vi "Write.vi"(2 "Element":T1, 3 "timeout in ms (-1)":i32, 4 "Close (F)":bool) -> (7 "EnclaveChannel":T2, 8 "Closed?":bool, 9 "timed out?":bool)   [LabVIEW 2022 SP3, in "Enclave.lvlib"]
doc: "Writes values directly to the Channel Wire. How the value is transferred will depend on what readers are connected to the Channel Wire. Writes will typically return quickly unless there are size bounded lossless readers attached to the Channel Wire that cause writes to block until those readers have space available."
uses:
  Enclave.lvlib
  ))Channel.ctl
  Element.ctl
  Operation.ctl
  Enclave/Enclave.lvclass/Enclave.ctl
  Enclave/Check Ready.vi
  Enclave/Enclave.lvclass
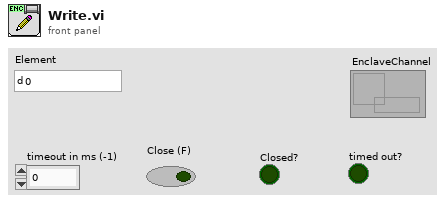
[diagram p1: front panel]
types:
  T1 = typedef "Enclave.lvlib/Element.ctl" = dbl
  T2 = typedef "Enclave.lvlib/))Channel.ctl" = refnum<queue>
  T3 = typedef "Enclave.lvlib/Operation.ctl" = enum16{"Get Core", "Init", "Close"}
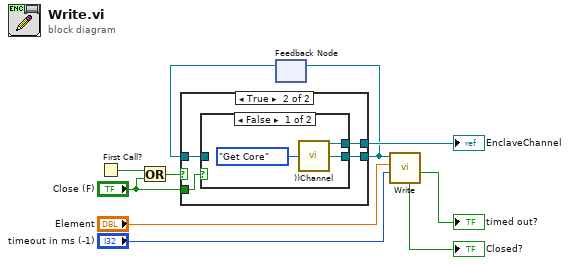
[diagram p0: block diagram]
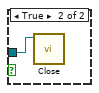
[diagram p3: hidden frame]
diagram:
  n1 = First Call?() -> (First Call?: T/F=w6:bool)
  n2 = Or(x=w6, y="Close (F)") -> (x .or. y?=w4:bool)
  n3 = feedback #1() -> (w10:refnum<class "Enclave.lvclass">)  [unwired: 1 in]
  n4 = case shown="True" w4 {
    tunnel: [_ w15] -> w5
    tunnel: [w11 w14] -> w2
    tunnel: w10 -> [w11 w12]
    tunnel: "Close (F)" -> [_ w13]
    frame False {
    }
    frame True {
      n5 = case shown="False" w13 {
        tunnel: [w18 _] -> w15
        tunnel: [w16 _] -> w14
        tunnel: w12 -> [_ w19]
        frame False {
          n6 = call "))Channel.vi"("Operation"=Operation."Get Core") -> ("EnclaveChannel out"=w18:T2, "Enclave"=w16:refnum<class "Enclave.lvclass">)  [unwired: 12 in, 1 out]
        }
        frame True {
          n7 = call "Close.vi"("Enclave in"=w19) -> ()  [unwired: 11 in]
        }
      }
    }
  }
  "EnclaveChannel" <- w5
  n8 = feedback-in #1(w2) -> ()
  n9 = call "Write.vi"("timeout in ms (-1)"="timeout in ms (-1)", "Element"="Element", "Enclave in"=w2) -> ("timed out?"=→"timed out?":bool, "Closed?"=→"Closed?":bool)  [unwired: 7 in]
